vi "PicoLogHRDLGetSingleExample.vi"() -> ()   [LabVIEW 2010]
panel:
  out "Unit Info":T1
  in  "Input type":i16(ring)=1 items=["Differential", "Single-Ended"]
  in  "Conversion time":i16(ring) items=["60ms", "100ms", "180ms", "340ms", "660ms"]
  in  "Voltage Range":i16(ring) items=["+/-2500mV", "+/-1250mV", "+/-625mV", "+/-312.5mV", "+/-156.25mV", "+/-78.125mV", "+/-39.0625mV"]
  out "Meter (mV)":dbl(knob)=-inf min=-39.0 max=39.0 scale=-2500.0..2500.0
  out "Over Range":i16 format="%016b"
  in  "Channel":i16=1 min=1 max=16 step=1
  in  "Mains Frequency":i16(ring) items=["50 Hz", "60 Hz"]
  in  "error in (no error)":errorcluster
  # "NOTES-\nNumber of channels-\nADC-20: 1 to 8\nADC-24: 1 to 16\n\nRange Voltage range Availability\n (0)    ±2500 mV        ADC-20 and ADC-24\n (1)    ±1250 mV        ADC-20 and ADC-24\n (2)    ±625 mV          ADC-24 only\n (3)    ±312.5 mV       ADC-24 only\n (4)    ±156.25 mV     ADC-24 only\n (5)    ±78.125 mV     ADC-24 only\n (6)    ±39.0625 mV   ADC-24 only"
  # "mV"
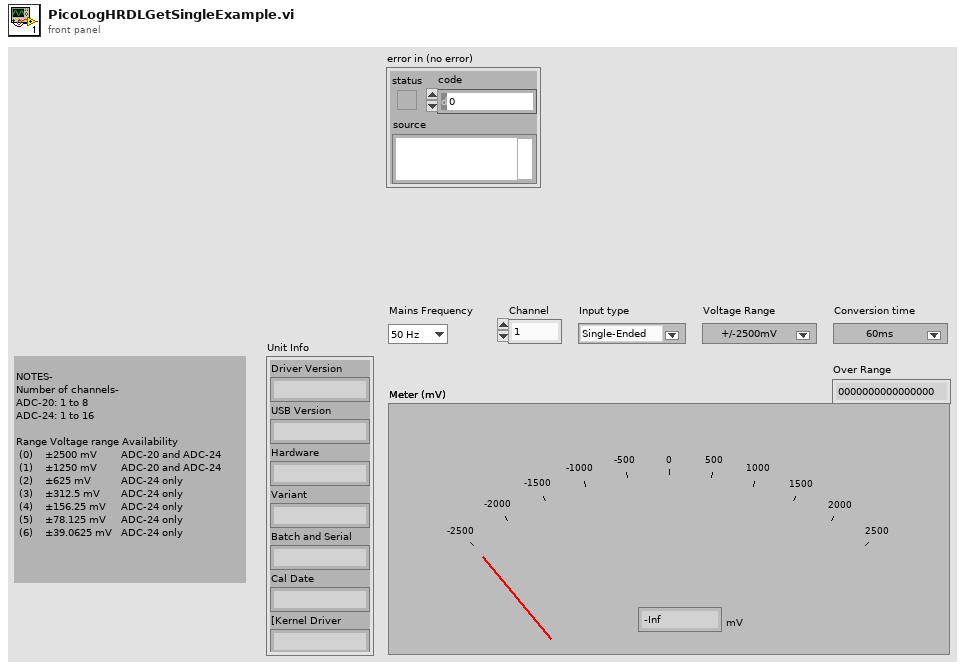
[diagram p1: front panel]
types:
  T1 = cluster{"Driver Version":string, "USB Version":string, "Hardware":string, "Variant":string, "Batch and Serial":string, "Cal Date":string, "[Kernel Driver":string, "[7]":string, "[8]":string, "[9]":string, "[10]":string, "[11]":string, "[12]":string, "[13]":string, "[14]":string}
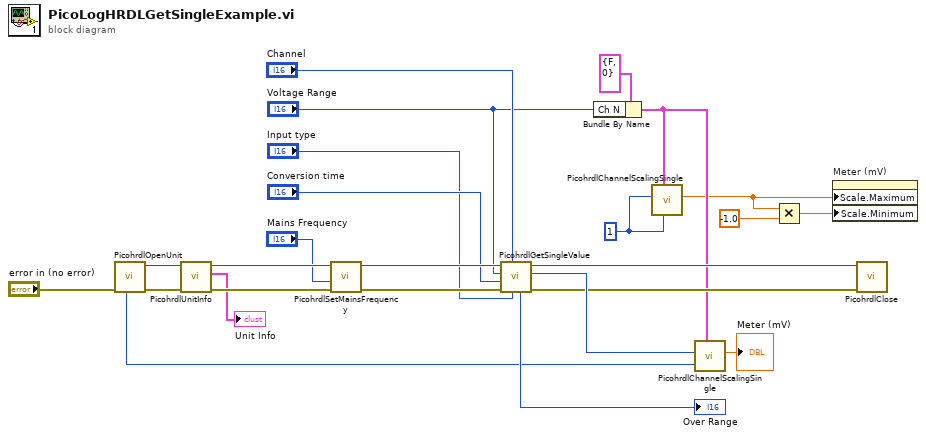
[diagram p0: block diagram]
diagram:
  w3 = 1 ("Max_adc")
  n1 = call "PicohrdlOpenUnit.vi"("error in (no error)"="error in (no error)") -> ("error out"=w20:errorcluster, "Handle out"=w19:i16, "maxAdc"=w1:i32)  [unwired: 7 in, 1 out]
  n2 = call "PicohrdlUnitInfo.vi"("error in (no error)"=w20, "handle in"=w19) -> ("error out"=w17:errorcluster, "Unit Info"=→"Unit Info":T1, "handle out"=w16:i16)  [unwired: 7 in]
  n3 = call "PicohrdlSetMainsFrequency.vi"("error in (no error)"=w17, "Mains Frequency"="Mains Frequency", "Handle in"=w16) -> ("error out"=w25:errorcluster, "Handle out"=w24:i16)  [unwired: 7 in]
  n4 = call "PicohrdlGetSingleValue.vi"("Single Ended"="Input type", "Channel in"="Channel", "error in (no error)"=w25, "Conversion"="Conversion time", "Voltage Range in"="Voltage Range", "handle in"=w24) -> ("error out"=w21:errorcluster, "value"=w23:i16, "Handle out"=w22:i16, "Over Voltage"=→"Over Range":i16)  [unwired: 2 in]
  n5 = Bundle By Name(cluster=cluster{bool, "Ch N":i16} {FALSE, "Ch N"=0} ("input cluster"), "Ch N"="Voltage Range") -> (w5:cluster{bool, "Ch N":i16})
  n6 = call "PicohrdlChannelScalingSingle.vi"("Max_adc"=w3, "Channel N"=w5, "DataIn"=w3) -> ("DataOut"=w4:dbl)  [unwired: 8 in]
  n7 = call "PicohrdlChannelScalingSingle.vi"("Max_adc"=w1, "Channel N"=w5, "DataIn"=w23) -> ("DataOut"=→"Meter (mV)":dbl)  [unwired: 8 in]
  n8 = Multiply(x=w4, y=-1.0) -> (x*y=w6:dbl)
  n9 = property on="Meter (mV)" class="Knob (strict)"("Scale.Maximum"=w4, "Scale.Minimum"=w6) -> ()  [unwired: 2 in, 2 out]
  n10 = call "PicohrdlClose.vi"("error in (no error)"=w21, "Handle in"=w22) -> ()  [unwired: 8 in, 2 out]
